vi "RPC Method helloworld_Greeter_SayHello.vi"(8 "error in (no error)":errorcluster, 11 "OOP Server in":refnum<class "Greeter.lvclass">) -> (0 "error out":errorcluster, 3 "OOP Server out":refnum<class "Greeter.lvclass">)   [LabVIEW 2019, in "helloworld_server.lvlib" / "Greeter.lvclass"]
uses:
  Greeter.lvclass
  Greeter.lvclass/Greeter.ctl
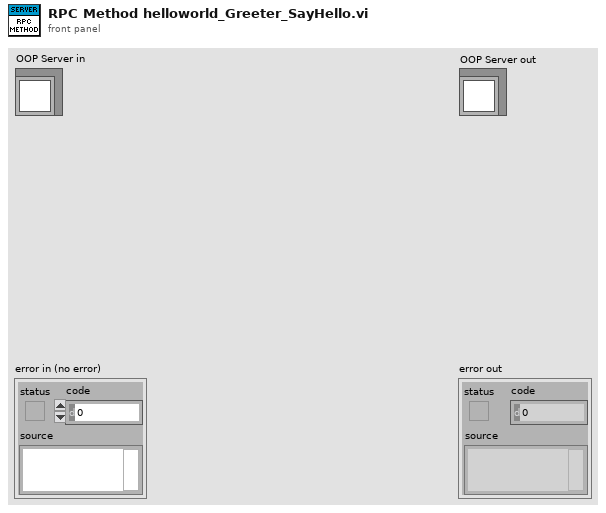
[diagram p1: front panel]
types:
  T1 = typedef "helloworld_server.lvlib/Greeter.lvclass/Server Internal UEs.ctl" = cluster{"helloworld_Greeter_SayHello Internal UE":refnum<user-event>}
  T2 = typedef "helloworld_server.lvlib/Greeter.lvclass/Server gRPC UEs.ctl" = cluster{"helloworld_Greeter_SayHello gRPC UE":refnum<user-event>}
  T3 = typedef "gprc-lvsupport-release.lvlib/grpcId.ctl" = u64
  T4 = typedef "helloworld_server.lvlib/helloworld_HelloRequest.ctl" = cluster{"name":string}
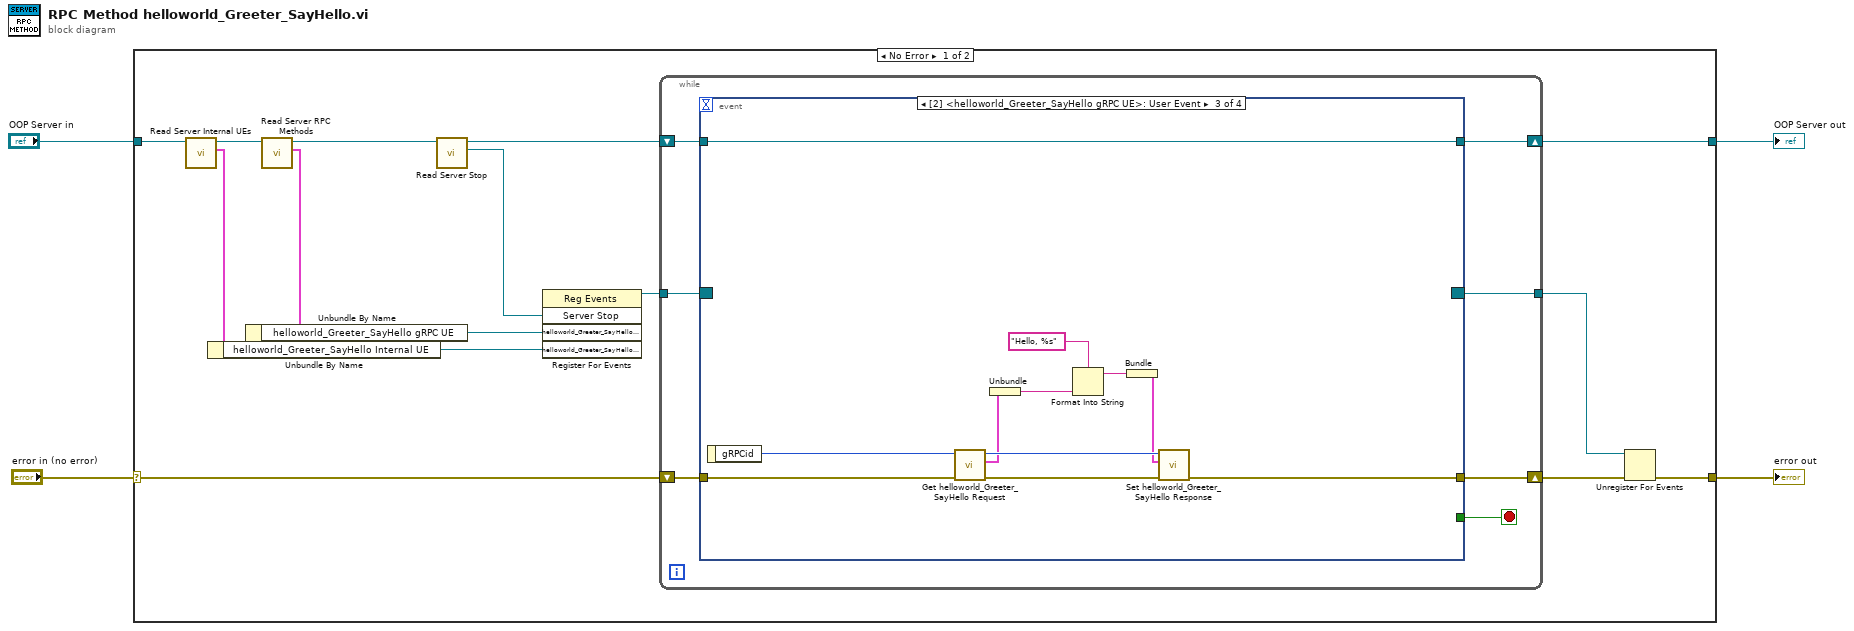
[diagram p0: block diagram]
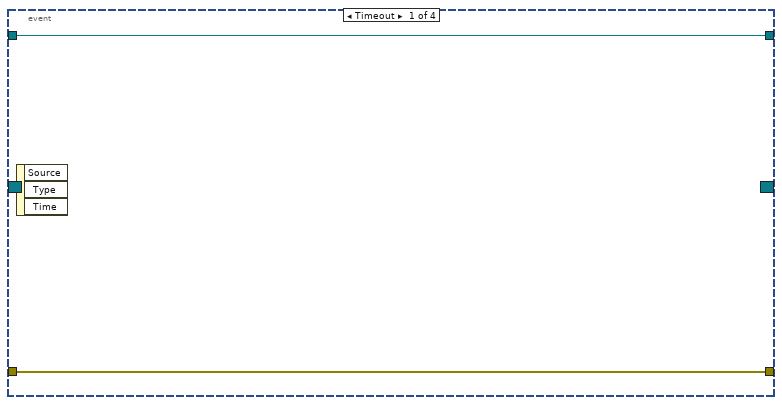
[diagram p2: hidden frame]
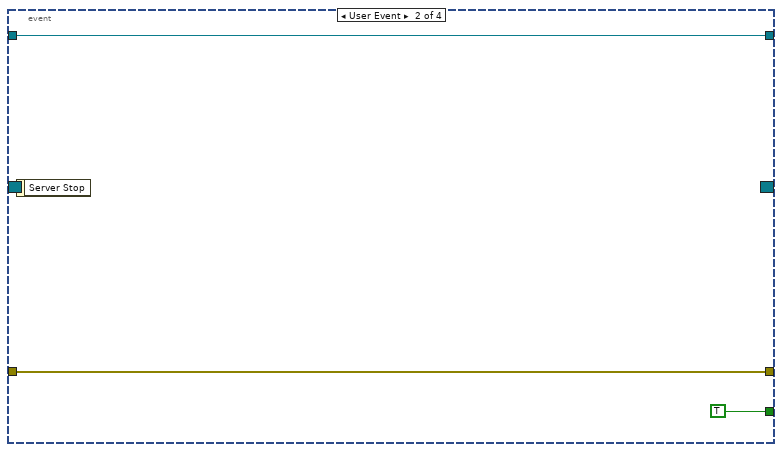
[diagram p3: hidden frame]
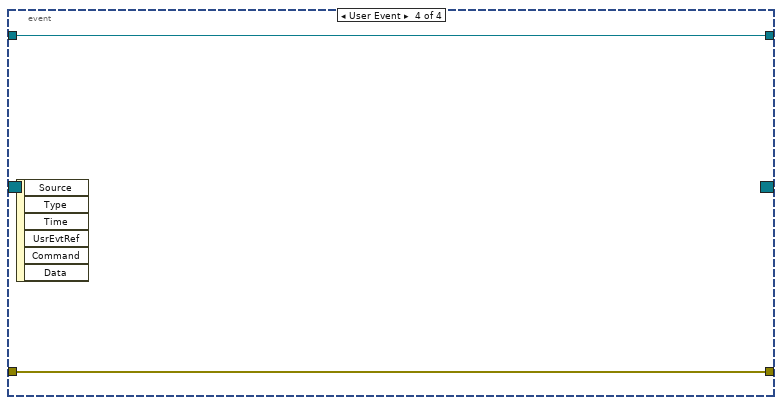
[diagram p4: hidden frame]
diagram:
  n1 = case shown="No Error" "error in (no error)" {
    selector: "error in (no error)" -> [w15 w46]
    tunnel: [w13 w46] -> w3
    tunnel: "OOP Server in" -> [w17 w45]
    tunnel: [w5 w45] -> w1
    frame No Error {
      n2 = call "Read Server Internal UEs.vi"("SignalGeneratorService in"=w17) -> ("Server Internal UEs"=w9:T1, "SignalGeneratorService out"=w16:refnum<class "Greeter.lvclass">)  [unwired: 8 in, 1 out]
      n3 = Unbundle By Name ("Unbundle Internal UE")(w9) -> ("helloworld_Greeter_SayHello Internal UE"=w8:refnum<user-event>)
      n4 = call "Read Server RPC Methods.vi"("SignalGeneratorService in"=w16) -> ("Server RPC Methods"=w11:T2, "SignalGeneratorService out"=w6:refnum<class "Greeter.lvclass">)  [unwired: 8 in, 1 out]
      n5 = Unbundle By Name ("Unbundle gRPC UE")(w11) -> ("helloworld_Greeter_SayHello gRPC UE"=w10:refnum<user-event>)
      n6 = call-dynamic "Read Server Stop.vi"("iService in"=w6) -> ("Server Stop"=w19:refnum<user-event>, "iService out"=w7:refnum<class "Greeter.lvclass">)  [unwired: 8 in, 1 out]
      n7 = register-events(w19, w10, w8) -> (reference out=w18:refnum<event-registration>)  [unwired: 2 in, 1 out]
      n8 = while {
        tunnel: w18 -> [w26]
        tunnel: [w22] -> w12
        shift-right: [w23] -> w14
        shift-left: w15 -> [w24]
        shift-right: [w20] -> w5
        shift-left: w7 -> [w21]
        stop <- w25 stop-if-true
        n9 = event "RPC Method Event Structure" shown="[2] <helloworld_Greeter_SayHello gRPC UE>: User Event" {
          selector: w26 -> [_ _ _ _]
          dyn-events: [_ _ _ _] -> w22
          timeout: _ -> [_ _ _ _]
          tunnel: [_ TRUE _ _] -> w25
          tunnel: w24 -> [w28 w30 w33 w44]
          tunnel: [w28 w30 w32 w44] -> w23
          tunnel: w21 -> [w27 w29 w42 w43]
          tunnel: [w27 w29 w42 w43] -> w20
          event Timeout {
            n10 = event-data() -> ()  [unwired: 1 in, 3 out]
          }
          event User Event {
            n11 = event-data() -> ()  [unwired: 1 in, 1 out]
          }
          event User Event {
            n12 = event-data() -> ("gRPCid"=w34:T3)  [unwired: 1 in]
            n13 = call "Get helloworld_Greeter_SayHello Request.vi"("error in (no error)"=w33, "gRPCid in"=w34) -> ("error out"=w40:errorcluster, "Message Data"=w39:T4, "gRPCid out"=w41:T3)  [unwired: 7 in]
            n14 = Unbundle(w39) -> ("name"=w37:string)
            n15 = Format Into String(format string="Hello, %s", w37) -> (resulting string=w35:string)  [unwired: 2 in, 1 out]
            n16 = Bundle(w35) -> (w38:cluster{string})  [unwired: 1 in]
            n17 = call "Set helloworld_Greeter_SayHello Response.vi"("error in (no error)"=w40, "Message Data"=w38, "gRPCid in"=w41) -> ("error out"=w32:errorcluster)  [unwired: 8 in]
          }
          event User Event {
            n18 = event-data() -> ()  [unwired: 1 in, 6 out]
          }
        }
      }
      n19 = Unregister For Events(event registration refnum=w12, error in=w14) -> (error out=w13:errorcluster)
    }
    frame Error {
    }
  }
  "error out" <- w3
  "OOP Server out" <- w1
